vi "Path AE.vi"(6 "Reverse? In (F)":bool, 7 "Path AE Action":T3, 8 "error in (no error)":errorcluster, 9 "Lookahead":dbl, 10 "Odometry":T1, 11 "Path Input":T2[](array[typedef])) -> (0 "error out":errorcluster, 1 "Finished?":bool, 2 "Distance":dbl, 3 "point":T2, 4 "Reverse? (F)":bool, 5 "index out":i32)   [LabVIEW 2019, in "Pure Pursuit.lvlib"]
uses:
  Pure Pursuit.lvlib
  Typedef/Path Point.ctl
  Typedef/Path AE Action.ctl
  Odometry/Typedef/Odometry.ctl
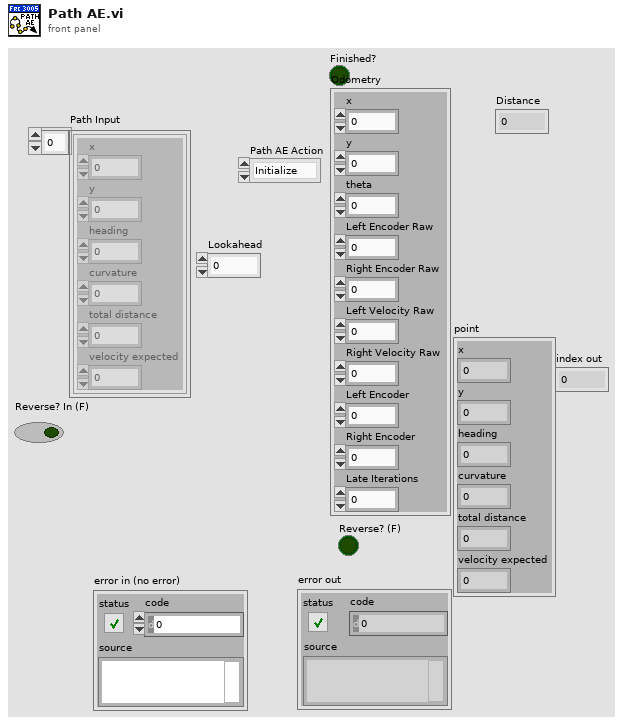
[diagram p1: front panel]
types:
  T1 = typedef "Odometry.ctl" = cluster{"x":dbl, "y":dbl, "theta":dbl, "Left Encoder Raw":i32, "Right Encoder Raw":i32, "Left Velocity Raw":i32, "Right Velocity Raw":i32, "Left Encoder":dbl, "Right Encoder":dbl, "Late Iterations":i16}
  T2 = typedef "Pure Pursuit.lvlib/Path Point.ctl" = cluster{"x":dbl, "y":dbl, "heading":dbl, "curvature":dbl, "total distance":dbl, "velocity expected":dbl}
  T3 = typedef "Pure Pursuit.lvlib/Path AE Action.ctl" = enum16{"Initialize", "Get Close Point", "Get Target Point", "Default", "Get Point", "Get Distance Remaining"}
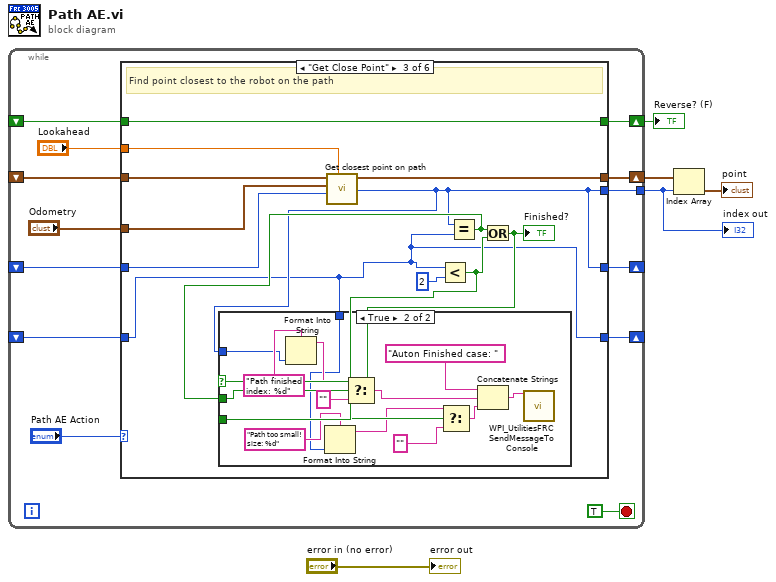
[diagram p0: block diagram]
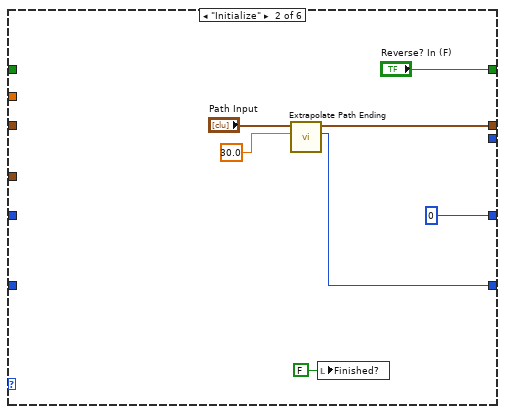
[diagram p3: hidden frame]
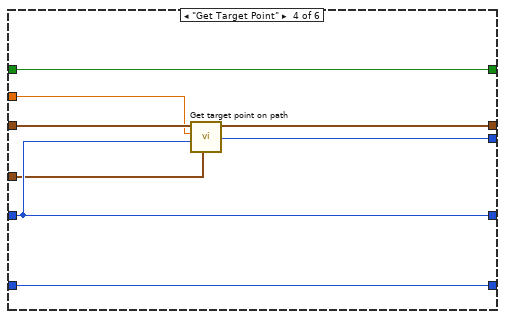
[diagram p5: hidden frame]
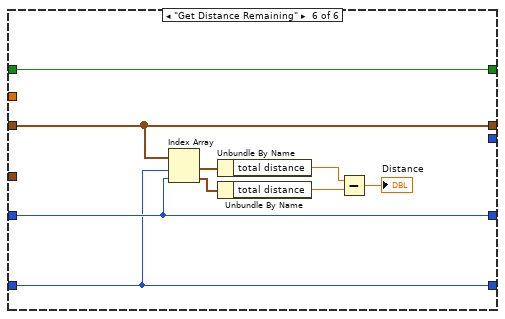
[diagram p7: hidden frame]
diagram:
  n1 = while {
    shift-right: [w16] -> w4
    shift-left: _ -> [w15]
    shift-right: [w14] -> _
    shift-left: _ -> [w13]
    tunnel: [w12] -> w3
    shift-right: [w9] -> w1
    shift-left: _ -> [w8]
    shift-right: [w7] -> _
    shift-left: _ -> [w6]
    stop <- TRUE stop-if-true
    n2 = case shown="\"Get Close Point\"" "Path AE Action" {
      tunnel: [w22 w26 w37 w63 w67 w70] -> w16
      tunnel: w15 -> [w22 _ w40 w62 w67 w70]
      tunnel: [w21 0 ("index") w31 w61 w66 w73] -> w14
      tunnel: w13 -> [w21 _ w41 w61 w66 w73]
      tunnel: "Odometry" -> [_ _ w39 w58 _ _]
      tunnel: [_ _ w31 w60 w66 _] -> w12
      tunnel: "Lookahead" -> [_ _ w38 w59 _ _]
      tunnel: [w20 "Reverse? In (F)" w35 w57 w65 w69] -> w9
      tunnel: w8 -> [w20 _ w35 w57 w65 w69]
      tunnel: [w19 w24 w30 w56 w64 w68] -> w7
      tunnel: w6 -> [w19 _ w30 w56 w64 w68]
      frame "Default", Default {
      }
      frame "Initialize" {
        n3 = call "Extrapolate Path Ending.vi"("Lookahead"=30.0, "Path in"="Path Input") -> ("End Point"=w24:i32, "Path out"=w26:T2[])  [unwired: 8 in]
        n4 = local write "Finished?"(FALSE ("Finished?")) -> ()
      }
      frame "Get Close Point" {
        # "Find point closest to the robot on the path"
        n5 = call "Get closest point on path.vi"("Lookahead"=w38, "index in"=w41, "Odometry"=w39, "Path in"=w40) -> ("index out"=w31:i32, "Path out"=w37:T2[])  [unwired: 6 in]
        n6 = Less?(x=w30, y=2) -> (x < y?=w33:bool)
        n7 = Equal?(x=w31, y=w30) -> (x = y?=w32:bool)
        n8 = Or(x=w32, y=w33) -> (x .or. y?=w34:bool)
        "Finished?" <- w34
        n9 = case shown="True" w34 {
          tunnel: w33 -> [_ w54]
          tunnel: w32 -> [_ w53]
          tunnel: w31 -> [_ w43]
          tunnel: w30 -> [_ w42]
          frame False {
          }
          frame True {
            n10 = Format Into String(format string="Path finished index: %d" ("f"), w43) -> (resulting string=w51:string)  [unwired: 2 in, 1 out]
            n11 = Format Into String(format string="Path too small! size: %d" ("f"), w42) -> (resulting string=w46:string)  [unwired: 2 in, 1 out]
            n12 = Select(t=w51, s=w53, f="") -> (s? t:f=w49:string)
            n13 = Select(t=w46, s=w54, f="") -> (s? t:f=w48:string)
            n14 = Concatenate Strings("Auton Finished case: " ("Message"), w49, w48) -> (w55:string)
            n15 = call <vilib>:"WPI_UtilitiesFRC SendMessageToConsole.vi"("Message"=w55) -> ()  [unwired: 14 in, 1 out]
          }
        }
      }
      frame "Get Target Point" {
        n16 = call "Get target point on path.vi"("Odometry"=w58, "index in"=w61, "Distance"=w59, "Path in"=w62) -> ("target index"=w60:i32, "Path out"=w63:T2[])  [unwired: 5 in, 1 out]
      }
      frame "Get Point" {
      }
      frame "Get Distance Remaining" {
        n17 = Index Array(array=w70, index #1=w68, index #2=w73) -> (element #1=w76:T2, element #2=w75:T2)
        n18 = Unbundle By Name(w76) -> ("total distance"=w72:dbl)
        n19 = Unbundle By Name(w75) -> ("total distance"=w74:dbl)
        n20 = Subtract(x=w72, y=w74) -> (x-y=→"Distance":dbl)
      }
    }
  }
  "Reverse? (F)" <- w1
  "index out" <- w3
  n21 = Index Array(array=w4, index=w3) -> (element=→"point":T2)
  "error out" <- "error in (no error)"
